vi "Maxi Gauge-RW Node Adress.vi"(7 "W/R":bool, 8 "Fehler (Eingang, kein Fehler)":errorcluster, 9 "Node adress 485-I Set":u8 max=31, 10 "Node address":i8=-1 min=-1 max=31 step=1, 11 "VISA-Ressource in":refnum<visa-resource-name>) -> (0 "Fehler (Ausgang)":errorcluster, 1 "Node adress 485-I Get":u8 max=31, 3 "VISA-Ressource out":refnum<visa-resource-name>)   [LabVIEW 2012, in "Maxi Gauge.lvlib"]
uses:
  Maxi Gauge.lvlib
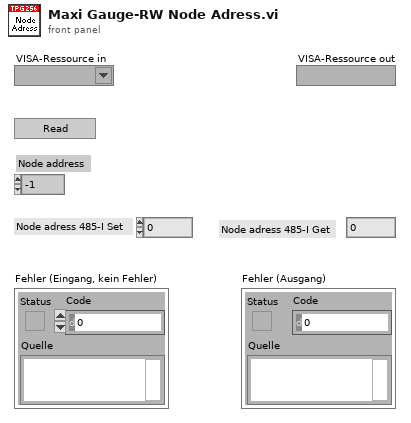
[diagram p1: front panel]
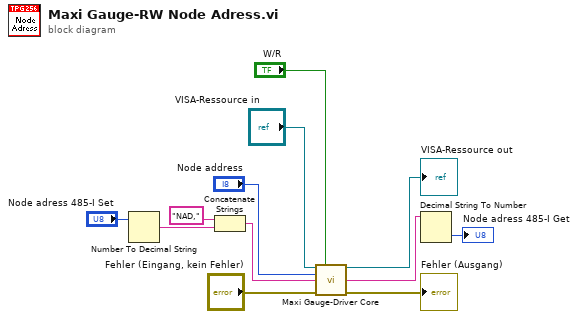
[diagram p0: block diagram]
diagram:
  n1 = Number To Decimal String(number="Node adress 485-I Set") -> (decimal integer string=w7:string)  [unwired: 1 in]
  n2 = Concatenate Strings("NAD," ("Command"), w7) -> (w5:string)
  n3 = call "Maxi Gauge-Driver Core.vi"("VISA-Ressource in"="VISA-Ressource in", "Write/Read"="W/R", "Node address"="Node address", "Command"=w5, "Fehler (Eingang)"="Fehler (Eingang, kein Fehler)") -> ("VISA-Ressource out"=→"VISA-Ressource out":refnum<visa-resource-name>, "String Out"=w6:string, "Fehler (Ausgang)"=→"Fehler (Ausgang)":errorcluster)  [unwired: 8 in]
  n4 = Decimal String To Number(string=w6) -> (number=→"Node adress 485-I Get":i32)  [unwired: 2 in, 1 out]
